vi "disconnect.vi"(8 "error in (no error)":errorcluster, 11 "Worker in":refnum<class "MQTT1.lvclass">) -> (0 "error out":errorcluster, 3 "Worker out":refnum<class "MQTT1.lvclass">)   [LabVIEW 2015, in "MQTT1.lvclass"]
uses:
  MQTT1.lvclass
  MQTT1.lvclass/MQTT1.ctl
  Libraries/mqtt Folder/src/class/mqtt/mqtt.lvclass
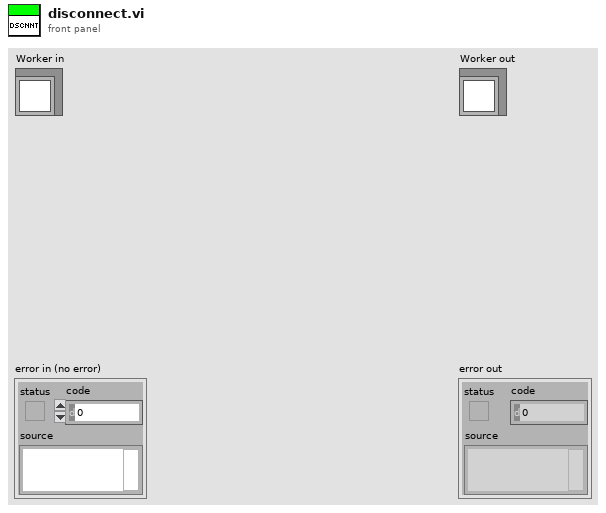
[diagram p1: front panel]
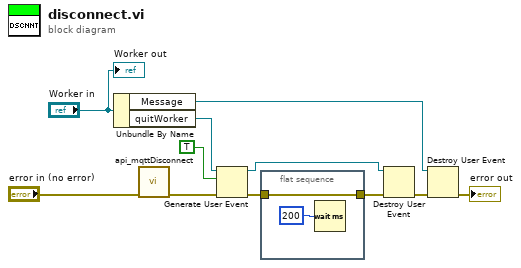
[diagram p0: block diagram]
diagram:
  n1 = Unbundle By Name("Worker in") -> ("Message"=w6:refnum<user-event>, "quitWorker"=w5:refnum<user-event>)
  n2 = call "api_mqttDisconnect.vi"("error in (no error)"="error in (no error)") -> ("error out"=w10:errorcluster)  [unwired: 13 in, 1 out]
  n3 = Generate User Event(user event=w5, event data cluster=TRUE ("event data"), error in=w10) -> (user event out=w1:refnum<user-event>, error out=w3:errorcluster)  [unwired: 1 in]
  n4 = flat-sequence {
    tunnel: [w12] -> w4
    tunnel: w3 -> [w12]
    frame #0 {
      n5 = Wait (ms)(milliseconds to wait=u32 200) -> ()  [unwired: 1 out]
    }
  }
  n6 = Destroy User Event(user event=w1, error in=w4) -> (error out=w8:errorcluster)
  n7 = Destroy User Event(user event=w6, error in=w8) -> (error out=→"error out":errorcluster)
  "Worker out" <- "Worker in"
